vi "Initialize.vi"(8 "error in (no error)":errorcluster, 9 "Node Config Version":string, 10 "Node Config":string, 11 "Node in":refnum<class "AMS Climate Chamber Template.lvclass"> caption="Timed Node in") -> (0 "error out":errorcluster, 1 "Init Output Version":string, 2 "Init Output":variant, 3 "Node out":refnum<class "AMS Climate Chamber Template.lvclass"> caption="Timed Node out")   [LabVIEW 2026, in "AMS Climate Chamber Template.lvlib" / "AMS Climate Chamber Template.lvclass"]
uses:
  AMS Climate Chamber Template.lvclass
  AMS Climate Chamber Template.lvclass/AMS Climate Chamber Template.ctl
  <vilib>/ADAS Replay HIL/Template Node/Plugin/Template Node/Template Node.lvclass
  <vilib>/ADAS Replay HIL/AdasHilServices/AdasHilChannelServices.lvlib
  <vilib>/ADAS Replay HIL/AdasHilServices/Server Mode.ctl
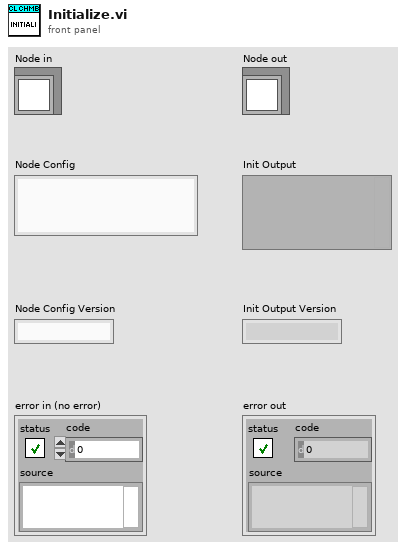
[diagram p1: front panel]
types:
  T1 = typedef "AdasHilChannelServices.lvlib/Server Mode.ctl" = enum8{"External Process", "In Process"}
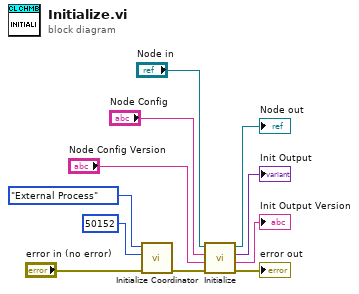
[diagram p0: block diagram]
diagram:
  n1 = call <vilib>:"Initialize Coordinator.vi"("error in"="error in (no error)", "Server Port"=50152, "Server Mode"=Server_Mode."External Process") -> ("error out"=w1:errorcluster)  [unwired: 8 in]
  n2 = call-parent "Initialize.vi"("error in (no error)"=w1, "Node Config Version"="Node Config Version", "Node Config"="Node Config", "Node in"="Node in") -> ("error out"=→"error out":errorcluster, "Init Output Version"=→"Init Output Version":string, "Init Output"=→"Init Output":variant, "Node out"=→"Node out":refnum<class "AMS Climate Chamber Template.lvclass">)  [unwired: 4 in]
